vi "convert tif to jpg.vi"() -> ()   [LabVIEW 2014]
uses:
  <vilib>/Utility/file.llb/Write To Spreadsheet File (DBL).vi
panel:
  out "Image":T1(plugin-control)
  in  "Correlation Time (s)":dbl
  in  "Max Voltage":dbl
  in  "Min Voltage":dbl
  in  "Frames":i32
  in  "Sigma":dbl
  in  "Offset Voltage":dbl
  out "Save Directory":path
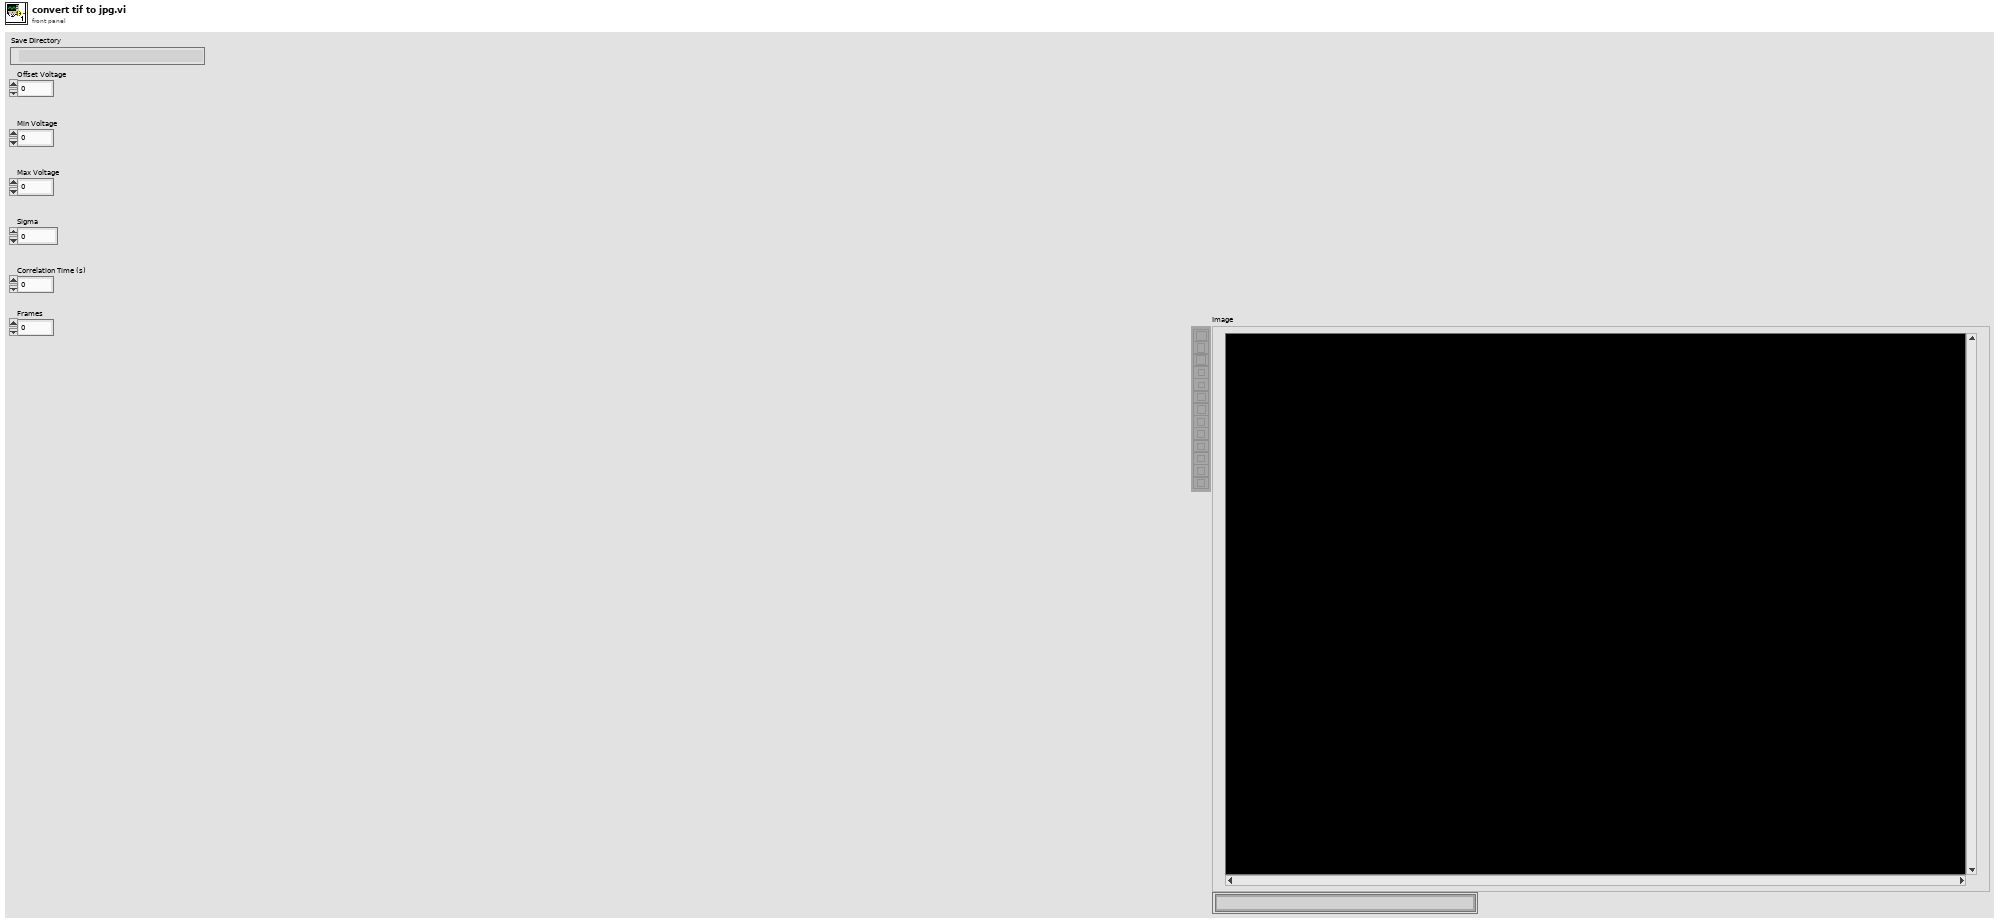
[diagram p1: front panel]
types:
  T1 = typedef "IMAQ Image.ctl" = refnum<image>
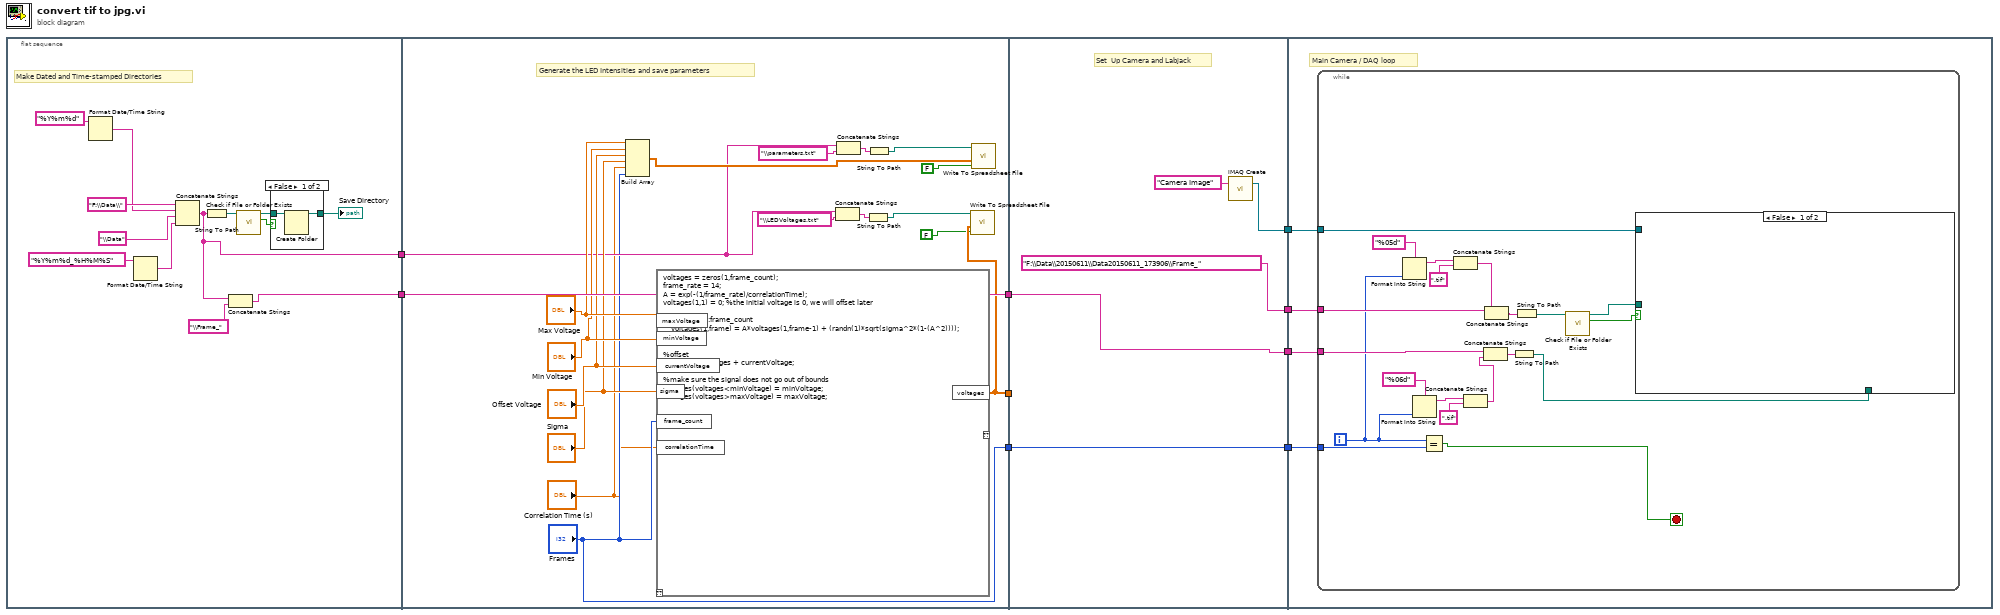
[diagram p0: block diagram]
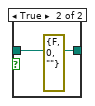
[diagram p2: hidden frame]
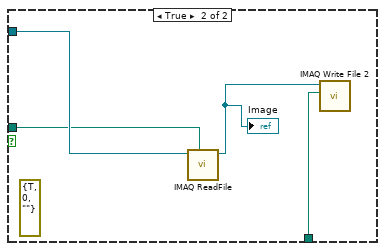
[diagram p3: hidden frame]
diagram:
  n1 = flat-sequence {
    tunnel: [w12] -> w4
    tunnel: [w10] -> w3
    tunnel: [w41] -> w8
    tunnel: [w39] -> w7
    tunnel: ["Frames"] -> w6
    tunnel: w3 -> [w28]
    tunnel: w4 -> [w41]
    tunnel: w8 -> [w45]
    tunnel: ["F:\\Data\\20150611\\Data20150611_173906\\Frame_"] -> w9
    tunnel: w7 -> [_]
    tunnel: w6 -> [w48]
    tunnel: [w48] -> w5
    tunnel: [w45] -> w2
    tunnel: [w46] -> w1
    tunnel: w2 -> [w50]
    tunnel: w5 -> [w51]
    tunnel: w9 -> [w52]
    tunnel: w1 -> [w49]
    frame #0 {
      # "Make Dated and Time-stamped Directories"
      n2 = Format Date/Time String(time format string (%c)="%Y%m%d") -> (date/time string=w13:string)  [unwired: 2 in]
      n3 = Format Date/Time String(time format string (%c)="%Y%m%d_%H%M%S") -> (date/time string=w17:string)  [unwired: 2 in]
      n4 = Concatenate Strings("F:\\Data\\", w13, "\\Data", w17) -> (w10:string)
      n5 = String To Path(string=w10) -> (path=w16:path)
      n6 = Concatenate Strings(w10, "\\Frame_") -> (w12:string)
      n7 = call <vilib>:"Check if File or Folder Exists.vi"("path"=w16) -> ("file or folder exists?"=w21:bool, "dup path"=w20:path)  [unwired: 8 in, 1 out]
      n8 = case shown="False" w21 {
        tunnel: [w23 w25] -> w15
        tunnel: w20 -> [w24 w25]
        frame False {
          n9 = Create Folder(path (use dialog)=w24) -> (created path=w23:path)  [unwired: 2 in, 2 out]
        }
        frame True {
          (unwired) errorcluster {"status"=FALSE, "code"=0, "source"=""} ("error out")
        }
      }
      "Save Directory" <- w15
    }
    frame #1 {
      # "Generate the LED Intensities and save parameters"
      n10 = Build Array("Max Voltage", "Min Voltage", "Offset Voltage", "Sigma", "Correlation Time (s)", "Frames") -> (w29:dbl[])
      n11 = script code="voltages = zeros(1,frame_count);\nframe_rate = 14;\nA = exp(-(1/frame_rate)/correlationTime);\nvoltages(1,1) = 0; %the initial voltage is 0, we will offset later\n\nfor frame = 2:frame_count\n    voltages(1,frame) = A*voltages(1,frame-1) + (randn(1)*sqrt(sigma^2*(1-(A^2))));\nend\n\n%offset\nvoltages = voltages + currentVoltage;\n\n%make sure the signal does not go out of bounds\nvoltages(voltages<minVoltage) = minVoltage;\nvoltages(voltages>maxVoltage) = maxVoltage;"("currentVoltage"="Offset Voltage", "frame_count"="Frames", "sigma"="Sigma", "minVoltage"="Min Voltage", "maxVoltage"="Max Voltage", "correlationTime"="Correlation Time (s)") -> ("voltages"=w39:dbl[])  [unwired: 1 in, 1 out]
      n12 = Concatenate Strings(w28, "\\LEDVoltages.txt") -> (w43:string)
      n13 = Concatenate Strings(w28, "\\parameters.txt") -> (w33:string)
      n14 = String To Path(string=w43) -> (path=w42:path)
      n15 = String To Path(string=w33) -> (path=w32:path)
      n16 = call-poly <vilib>:"Write To Spreadsheet File.vi"("append to file? (new file:F)"=FALSE, "1D data"=w39, "file path (dialog if empty)"=w42) -> ()  [unwired: 5 in, 1 out]
      n17 = call-poly <vilib>:"Write To Spreadsheet File.vi"("append to file? (new file:F)"=FALSE, "1D data"=w29, "file path (dialog if empty)"=w32) -> ()  [unwired: 5 in, 1 out]
    }
    frame #2 {
      # "Set  Up Camera and Labjack"
      n18 = call "IMAQ Create"("Image Name"="Camera Image") -> ("New Image"=w46:T1)  [unwired: 4 in, 1 out]
    }
    frame #3 {
      # "Main Camera / DAQ loop"
      n19 = while {
        tunnel: w52 -> [w67]
        tunnel: w51 -> [w69]
        tunnel: w50 -> [w65]
        tunnel: w49 -> [w59]
        i -> [w54]
        stop <- w68 stop-if-true
        n20 = Format Into String(format string="%05d" ("string"), w54) -> (resulting string=w71:string)  [unwired: 2 in, 1 out]
        n21 = Format Into String(format string="%06d" ("string"), w54) -> (resulting string=w56:string)  [unwired: 2 in, 1 out]
        n22 = Equal?(x=w54, y=w69) -> (x = y?=w68:bool)
        n23 = Concatenate Strings(w71, ".tif" ("string")) -> (w64:string)
        n24 = Concatenate Strings(w56, ".tif" ("string")) -> (w53:string)
        n25 = Concatenate Strings(w65, w53) -> (w63:string)
        n26 = Concatenate Strings(w67, w64) -> (w66:string)
        n27 = String To Path(string=w63) -> (path=w58:path)
        n28 = String To Path(string=w66) -> (path=w60:path)
        n29 = call <vilib>:"Check if File or Folder Exists.vi"("path"=w60) -> ("file or folder exists?"=w62:bool, "dup path"=w61:path)  [unwired: 8 in, 1 out]
        n30 = case shown="False" w62 {
          tunnel: w61 -> [_ w74]
          tunnel: w59 -> [_ w76]
          tunnel: w58 -> [_ w75]
          frame False {
          }
          frame True {
            (unwired) errorcluster {"status"=TRUE, "code"=0, "source"=""} ("error out")
            n31 = call "IMAQ ReadFile"("File Path"=w74, "Image"=w76) -> ("Image Out"=w73:T1)  [unwired: 5 in, 4 out]
            "Image" <- w73
            n32 = call-poly "IMAQ Write File 2"("File Path"=w75, "Image"=w73) -> ()  [unwired: 8 in, 2 out]
          }
        }
      }
    }
  }
